vi "DrawLine.vi"(8 "Line Width (px)":u8=1, 9 "Color":u32(colorbox), 10 "Line Endpoints":cluster{dbl, dbl}[](array[cluster]), 11 "Image":T1) -> (3 "Image Out":T1)   [LabVIEW 2017, in "ArgosLib.lvlib"]
uses:
  <vilib>/vision/Image Controls.llb/IMAQ Image.ctl
  ArgosLib.lvlib
  <vilib>/vision/NI_Vision_Development_Module.lvlib
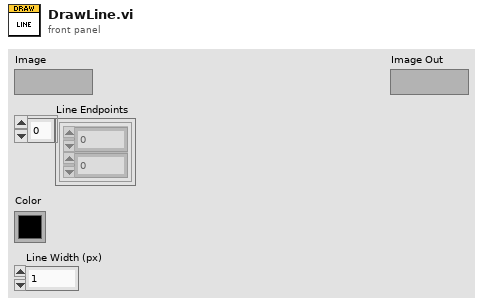
[diagram p1: front panel]
types:
  T1 = typedef "IMAQ Image.ctl" = refnum<image>
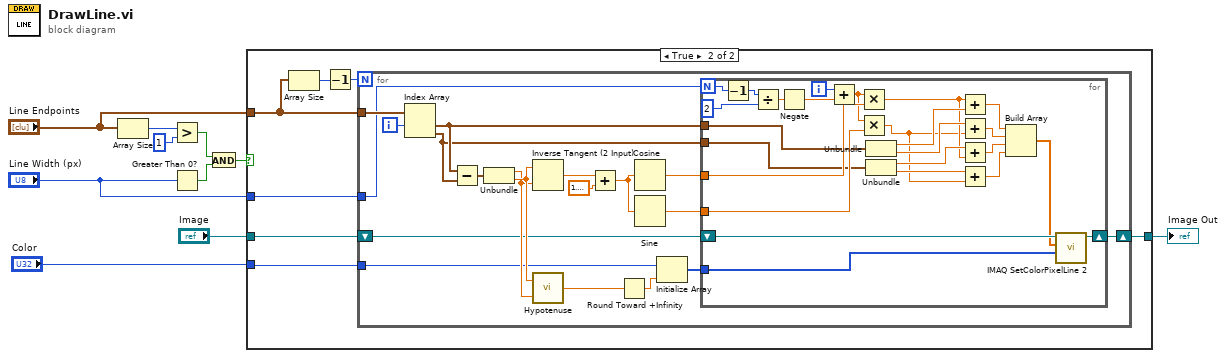
[diagram p0: block diagram]
diagram:
  n1 = Array Size(array="Line Endpoints") -> (size(s)=w8:i32)
  n2 = Greater?(x=w8, y=1) -> (0:w6:bool)
  n3 = Greater Than 0?(x="Line Width (px)") -> (x > 0?=w5:bool)
  n4 = And(x=w6, y=w5) -> (x .and. y?=w4:bool)
  n5 = case shown="True" w4 {
    tunnel: "Image" -> [w11 w13]
    tunnel: [w11 w12] -> w9
    tunnel: "Color" -> [_ w14]
    tunnel: "Line Width (px)" -> [_ w15]
    tunnel: "Line Endpoints" -> [_ w16]
    frame False {
    }
    frame True {
      n6 = Array Size(array=w16) -> (size(s)=w18:i32)
      n7 = Decrement(x=w18) -> (x-1=w17:i32)
      n8 = for {
        N: w17 -> [_]
        tunnel: w16 -> [w37]
        tunnel: w15 -> [w35]
        tunnel: w14 -> [w24]
        shift-right: [w21] -> w12
        shift-left: w13 -> [w22]
        i -> [w36]
        n9 = Index Array(array=w37, index #1=w36) -> (element #1=w34:cluster{dbl, dbl}, element #2=w33:cluster{dbl, dbl})  [unwired: 1 in]
        n10 = Subtract(x=w34, y=w33) -> (x-y=w32:cluster{dbl, dbl})
        n11 = Unbundle(w32) -> (w27:dbl, w28:dbl)
        n12 = Inverse Tangent (2 Input)(1:w27, 2:w28) -> (0:w29:dbl)
        n13 = call "Hypotenuse.vi"("Y"=w27, "X"=w28) -> ("Hypotenuse"=w26:dbl)
        n14 = Add(x=w29, y=1.5707963267948966) -> (x+y=w20:dbl)
        n15 = Round Toward +Infinity(x=w26) -> (ceil(x): smallest int >= x=w25:dbl)
        n16 = Cosine(x=w20) -> (cos(x)=w31:dbl)
        n17 = Sine(x=w20) -> (sin(x)=w30:dbl)
        n18 = Initialize Array(w24, w25) -> (w23:u32[])
        n19 = for {
          N: w35 -> [w62]
          tunnel: w34 -> [w51]
          tunnel: w33 -> [w50]
          tunnel: w31 -> [w57]
          tunnel: w30 -> [w55]
          tunnel: w23 -> [w54]
          shift-right: [w52] -> w21
          shift-left: w22 -> [w53]
          i -> [w59]
          n20 = Decrement(x=w62) -> (x-1=w60:i32)
          n21 = Divide(x=w60, y=2) -> (x/y=w58:dbl)
          n22 = Negate(x=w58) -> (-x=w38:dbl)
          n23 = Add(x=w59, y=w38) -> (x+y=w56:dbl)
          n24 = Multiply(x=w56, y=w57) -> (x*y=w40:dbl)
          n25 = Multiply(x=w56, y=w55) -> (x*y=w39:dbl)
          n26 = Unbundle(w51) -> (w49:dbl, w47:dbl)
          n27 = Unbundle(w50) -> (w48:dbl, w46:dbl)
          n28 = Add(x=w40, y=w49) -> (x+y=w45:dbl)
          n29 = Add(x=w47, y=w39) -> (x+y=w44:dbl)
          n30 = Add(x=w48, y=w40) -> (x+y=w42:dbl)
          n31 = Add(x=w46, y=w39) -> (x+y=w43:dbl)
          n32 = Build Array(w45, w44, w42, w43) -> (w41:dbl[])
          n33 = call "IMAQ SetColorPixelLine 2"("Pixels Line (U32)"=w54, "Line Coordinates"=w41, "Image"=w53) -> ("Image Out"=w52:T1)  [unwired: 7 in, 1 out]
        }
      }
    }
  }
  "Image Out" <- w9
